vi "Sincronizza DB motori.vi"(11 "Slide 2":refnum<vi>) -> (0 "error out":errorcluster)   [LabVIEW 2019]
uses:
  <vilib>/Utility/file.llb/Read From Spreadsheet File (string).vi
  <vilib>/addons/database/Connection.llb/DB Tools Open Connec (String).vi
  <vilib>/addons/database/Connection.llb/Conn Execute.vi
  <vilib>/addons/database/Recordset.llb/Rec Fetch Recordset Data (R).vi
  <vilib>/addons/database/_DB Variant To Data/Database Variant To Data.xnode
  <vilib>/addons/database/NI_Database_API.lvlib
panel:
  out "spreadsheet string":string
  out "concatenated string":string
  in  "error in (no error) 2":errorcluster
  out "data":string[][](array[string])
  in  "error in (no error)":errorcluster
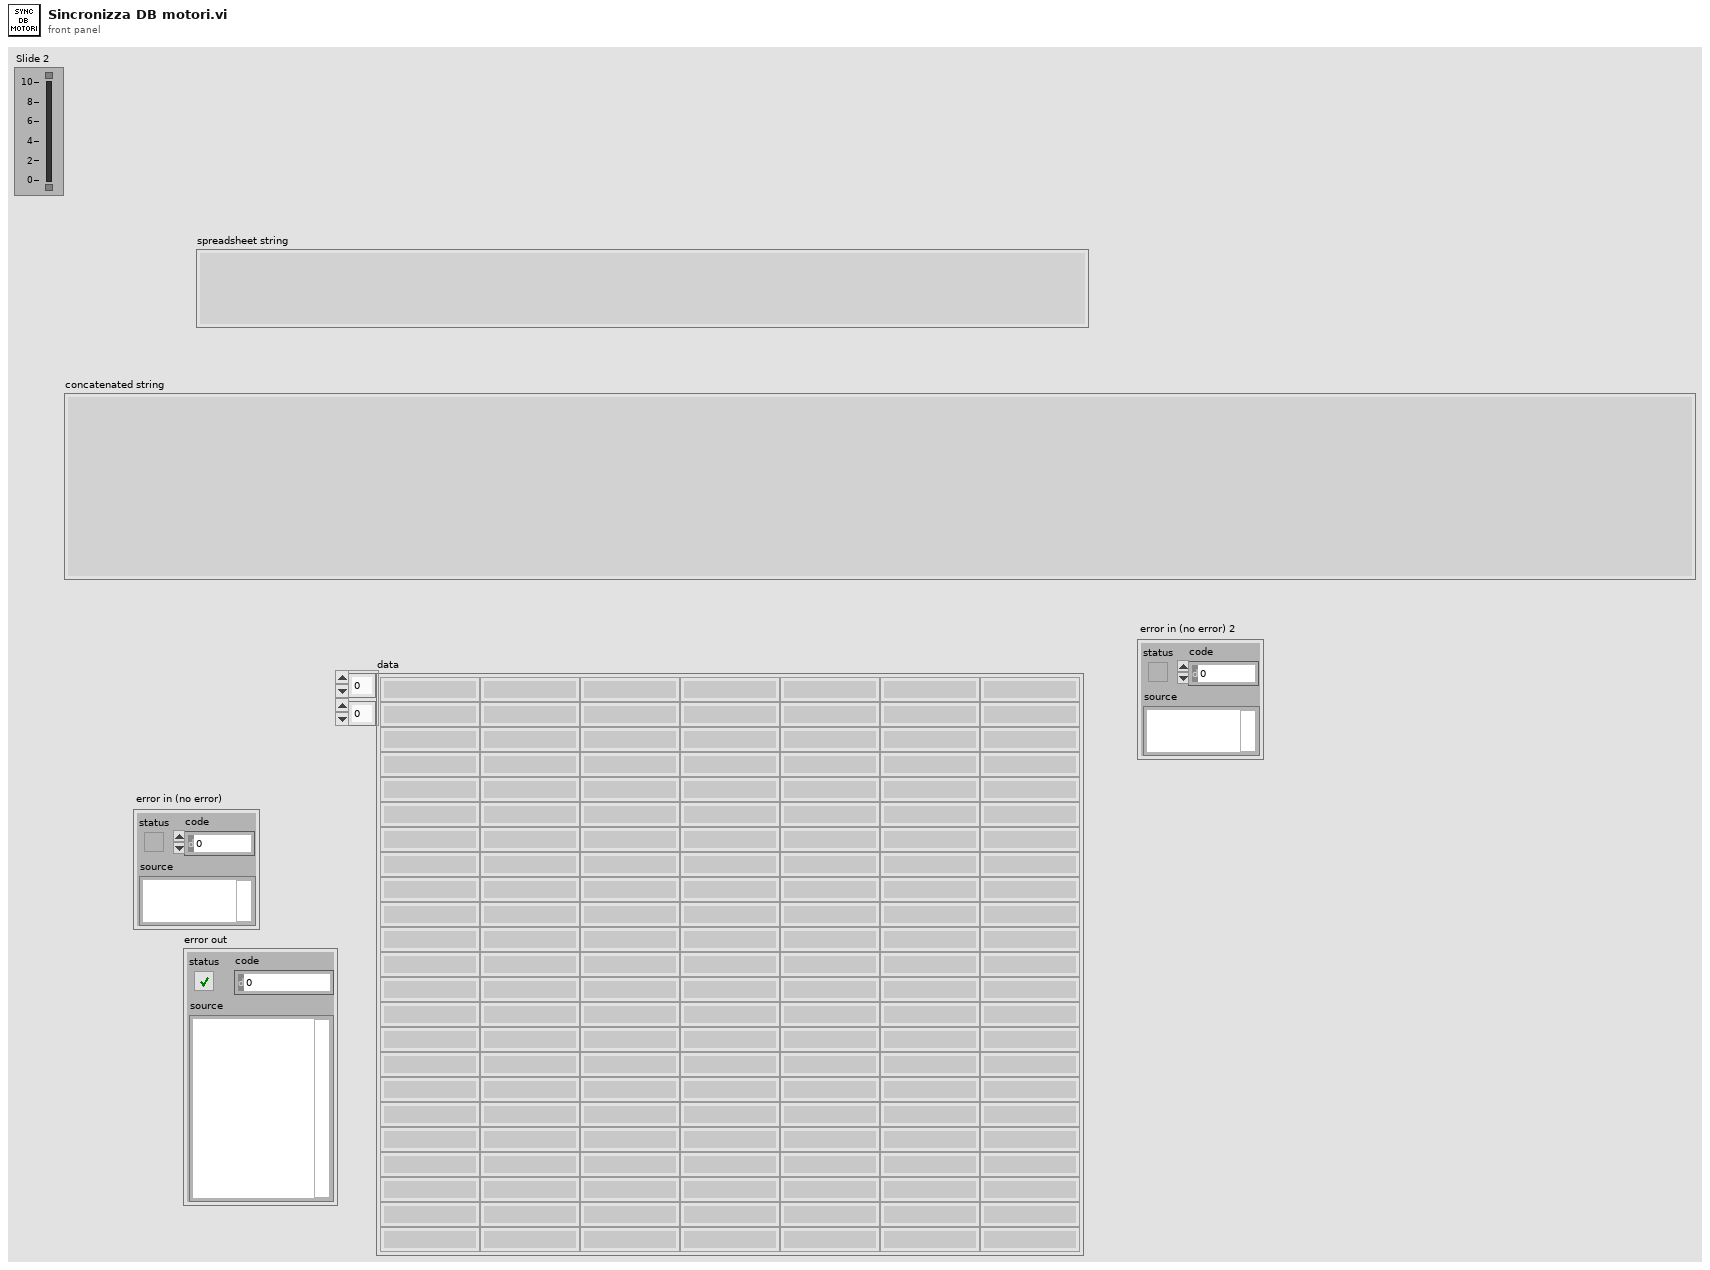
[diagram p1: front panel]
types:
  T1 = typedef "NI_Database_API.lvlib/Conn ObjectReference.ctl" = refnum<k1>
  T2 = typedef "NI_Database_API.lvlib/Rec ObjectReference.ctl" = refnum<k1>
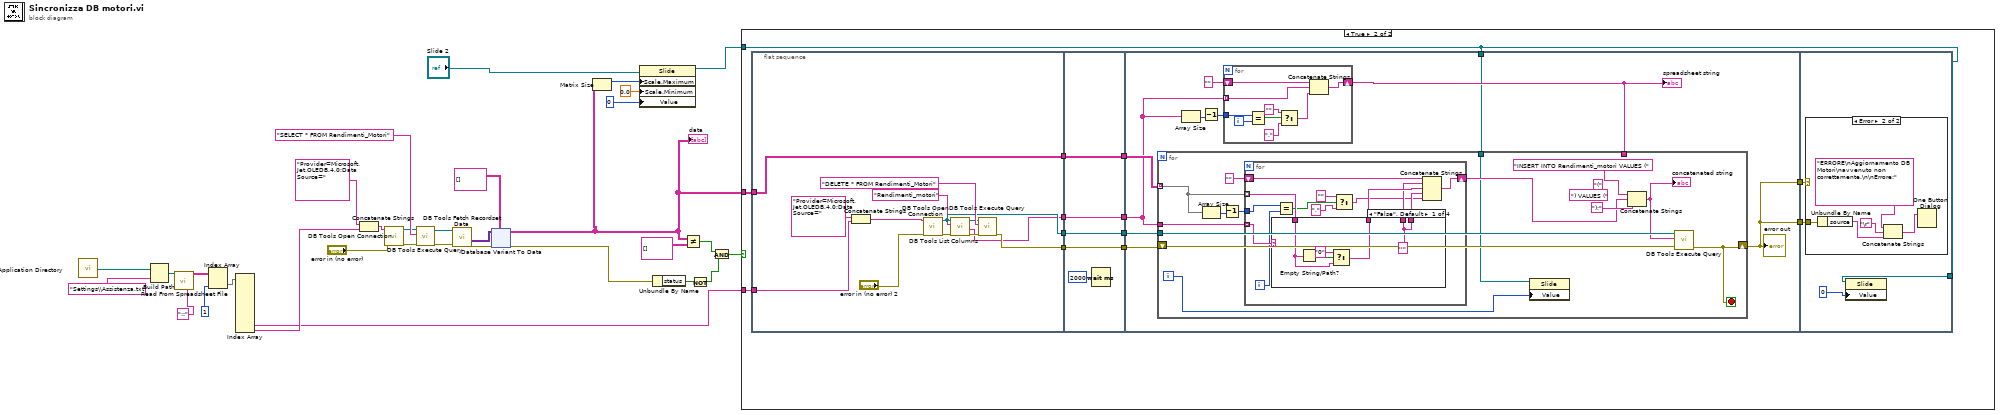
[diagram p0: block diagram]
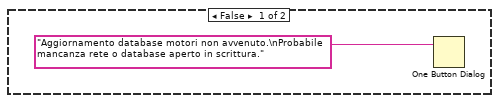
[diagram p2: hidden frame]
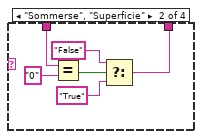
[diagram p3: hidden frame]
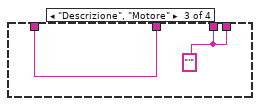
[diagram p4: hidden frame]
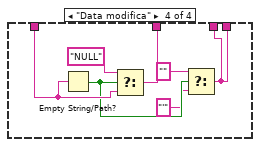
[diagram p5: hidden frame]
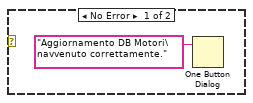
[diagram p6: hidden frame]
diagram:
  n1 = call <vilib>:"Application Directory.vi"() -> ("Application Directory"=w9:path)
  n2 = Build Path(base path=w9, name or relative path="Settings\\Assistenza.txt") -> (appended path=w7:path)
  n3 = call-poly <vilib>:"Read From Spreadsheet File.vi"("delimiter (\\t)"="::" ("delimiter (\\t)"), "file path (dialog if empty)"=w7) -> ("all rows"=w6:string[][])  [unwired: 5 in, 4 out]
  n4 = Index Array(array=w6, index (col)=1 ("disabled index (col)")) -> (element=w4:string[])  [unwired: 1 in]
  n5 = Index Array(array=w4) -> (element #9=w1:string, element #10=w2:string)  [unwired: 10 in, 8 out]
  n6 = Concatenate Strings("Provider=Microsoft.Jet.OLEDB.4.0;Data Source=" ("userID"), w2) -> (w31:string)
  n7 = call-poly <vilib>:"DB Tools Open Connection.vi"("error in (no error)"="error in (no error)", "connection information"=w31) -> ("error out"=w29:errorcluster, "connection reference"=w17:T1)  [unwired: 6 in]
  n8 = call-poly <vilib>:"DB Tools Execute Query.vi"("error in (no error)"=w29, "SQL query"="SELECT * FROM Rendimenti_Motori", "connection reference"=w17) -> ("error out"=w27:errorcluster, "recordset reference"=w16:T2)  [unwired: 5 in]
  n9 = call-poly <vilib>:"DB Tools Fetch Recordset Data.vi"("error in (no error)"=w27, "recordset reference"=w16) -> ("error out"=w26:errorcluster, "recordset data"=w25:variant[][])  [unwired: 3 in, 1 out]
  n10 = xnode "Database Variant To Data"("database variant"=w25, "error in (no error)"=w26, "type"=string[][] []) -> ("data"=w15:string[][], "error out"=w18:errorcluster)
  "data" <- w15
  n11 = Matrix Size(0:w15) -> (1:w14:i32)  [unwired: 1 out]
  n12 = property class="Slide"(reference="Slide 2", "Scale.Maximum"=w14, "Scale.Minimum"=0.0 ("Scale.Range:Minimum"), "Value"=u8 0) -> (reference out=w11:refnum<vi>)  [unwired: 1 in, 1 out]
  n13 = Unbundle By Name(w18) -> ("status"=w23:bool)
  n14 = Not Equal?(x=w15, y=string[][] []) -> (x != y?=w20:bool)
  n15 = Not(x=w23) -> (.not. x?=w21:bool)
  n16 = And(x=w20, y=w21) -> (x .and. y?=w19:bool)
  n17 = case shown="True" w19 {
    tunnel: w15 -> [_ w40]
    tunnel: w11 -> [_ w35]
    tunnel: w1 -> [_ w34]
    frame False {
      n18 = One Button Dialog(message="Aggiornamento database motori non avvenuto.\nProbabile mancanza rete o database aperto in scrittura.") -> ()  [unwired: 1 in, 1 out]
    }
    frame True {
      n19 = flat-sequence {
        tunnel: [w52] -> w46
        tunnel: [w55] -> w45
        tunnel: [w54] -> w41
        tunnel: w40 -> [w54]
        tunnel: [w50] -> w38
        tunnel: w34 -> [w47]
        tunnel: w46 -> [w63]
        tunnel: w45 -> [w62]
        tunnel: [w63] -> w44
        tunnel: [w62] -> w43
        tunnel: [w61] -> w42
        tunnel: w41 -> [w61]
        tunnel: [w60] -> w39
        tunnel: w38 -> [w60]
        tunnel: w44 -> [w66]
        tunnel: w43 -> [w74]
        tunnel: w42 -> [w73]
        tunnel: w39 -> [w68]
        tunnel: w35 -> [w67]
        tunnel: [w65] -> w37
        tunnel: [w65] -> w36
        tunnel: w37 -> [w134]
        tunnel: w36 -> [w133]
        tunnel: w35 -> [w132]
        frame #0 {
          n20 = Concatenate Strings("Provider=Microsoft.Jet.OLEDB.4.0;Data Source=" ("userID"), w47) -> (w57:string)
          n21 = call-poly <vilib>:"DB Tools Open Connection.vi"("error in (no error)"="error in (no error) 2", "connection information"=w57) -> ("error out"=w48:errorcluster, "connection reference"=w52:T1)  [unwired: 6 in]
          n22 = call <vilib>:"DB Tools List Columns.vi"("error in (no error)"=w48, "table"="Rendimenti_motori", "connection reference"=w52) -> ("error out"=w51:errorcluster, "columns"=w50:string[], "connection reference out"=w53:T1)  [unwired: 1 in, 1 out]
          n23 = call-poly <vilib>:"DB Tools Execute Query.vi"("error in (no error)"=w51, "SQL query"="DELETE * FROM Rendimenti_Motori", "connection reference"=w53) -> ("error out"=w55:errorcluster)  [unwired: 5 in, 1 out]
        }
        frame #1 {
          n24 = Wait (ms)(milliseconds to wait=u32 2000) -> ()  [unwired: 1 out]
        }
        frame #2 {
          n25 = Array Size(array=w68) -> (size(s)=w69:i32)
          n26 = Decrement(x=w69) -> (x-1=w71:i32)
          n27 = for {
            tunnel: w68 -> [w81] mode=indexing
            shift-right: [w82] -> w70
            shift-left: "" -> [w83]
            tunnel: w71 -> [w80]
            i -> [w79]
            n28 = Equal?(x=w80, y=w79) -> (x = y?=w78:bool)
            n29 = Select(t="" ("string"), s=w78, f="," ("t")) -> (s? t:f=w77:string)
            n30 = Concatenate Strings(w83, w81, w77) -> (w82:string)
          }
          "spreadsheet string" <- w70
          n31 = for {
            tunnel: w66 -> [w97]
            shift-right: [w84] -> w65
            shift-left: w74 -> [w96]
            tunnel: w73 -> [w90] mode=indexing
            tunnel: w70 -> [_]
            tunnel: w68 -> [w88]
            tunnel: w67 -> [w85]
            i -> [w86]
            stop <- w84 stop-if-true
            (unwired) ") VALUES (" ("string")
            (unwired) "(" ("string")
            n32 = Array Size(array=w90) -> (size(s)=w92:i32)
            n33 = Decrement(x=w92) -> (x-1=w93:i32)
            n34 = for {
              tunnel: w90 -> [w107] mode=indexing
              shift-right: [w109] -> w89
              shift-left: "" -> [w110]
              tunnel: w93 -> [w102]
              tunnel: w88 -> [w108] mode=indexing
              i -> [w103]
              n35 = case shown="\"False\", Default" w108 {
                tunnel: w107 -> [w114 w117 w122 w128]
                tunnel: [w112 w116 w122 w129] -> w106
                tunnel: [w111 _ w123 w125] -> w105
                tunnel: [w111 _ w123 w125] -> w104
                frame "False", Default {
                  w111 = "'" ("t")
                  n36 = Empty String/Path?(string/path=w114) -> (empty?=w115:bool)
                  n37 = Select(t="0", s=w115, f=w114) -> (s? t:f=w112:string)
                }
                frame "Sommerse", "Superficie" {
                  n38 = Equal?(x=w117, y="0") -> (x = y?=w120:bool)
                  n39 = Select(t="False" ("string"), s=w120, f="True" ("string")) -> (s? t:f=w116:string)
                }
                frame "Descrizione", "Motore" {
                  w123 = "'" ("string")
                }
                frame "Data modifica" {
                  n40 = Empty String/Path?(string/path=w128) -> (empty?=w127:bool)
                  n41 = Select(t="NULL", s=w127, f=w128) -> (s? t:f=w129:string)
                  n42 = Select(t="", s=w127, f="'" ("t")) -> (s? t:f=w125:string)
                }
              }
              n43 = Equal?(x=w102, y=w103) -> (x = y?=w101:bool)
              n44 = Select(t="", s=w101, f="," ("string")) -> (s? t:f=w99:string)
              n45 = Concatenate Strings(w110, w105, w106, w104, w99) -> (w109:string)
            }
            n46 = property class="Slide"(reference=w85, "Value"=w86) -> ()  [unwired: 1 in, 2 out]
            n47 = Concatenate Strings("INSERT INTO Rendimenti_motori VALUES (" ("string"), w89, ");" ("string")) -> (w95:string)
            "concatenated string" <- w95
            n48 = call-poly <vilib>:"DB Tools Execute Query.vi"("error in (no error)"=w96, "SQL query"=w95, "connection reference"=w97) -> ("error out"=w84:errorcluster)  [unwired: 5 in, 1 out]
          }
          "error out" <- w65
        }
        frame #3 {
          n49 = case shown="Error" w134 {
            tunnel: w133 -> [_ w140]
            frame No Error {
              n50 = One Button Dialog(message="Aggiornamento DB Motori\navvenuto correttamente.") -> ()  [unwired: 1 in, 1 out]
            }
            frame Error {
              n51 = Unbundle By Name(w140) -> ("source"=w138:string)
              n52 = Concatenate Strings("ERRORE\nAggiornamento DB Motori\navvenuto non correttamente.\n\nErrore:" ("message"), "\r", w138) -> (w136:string)
              n53 = One Button Dialog(message=w136) -> ()  [unwired: 1 in, 1 out]
            }
          }
          n54 = property class="Slide"(reference=w132, "Value"=0) -> ()  [unwired: 1 in, 2 out]
        }
      }
    }
  }
